vi "Erase color.vi"(8 "error in (no error)":errorcluster, 11 "Control-Client in":refnum<class "Control-Client.lvclass">) -> (0 "error out":errorcluster, 3 "Control-Client out":refnum<class "Control-Client.lvclass">)   [LabVIEW 2015, in "Control-Client.lvclass"]
uses:
  Control-Client.lvclass
  Control-Client.lvclass/Control-Client.ctl
  methods/Read Group #.vi
  Experiments/Experiments_group.lvclass
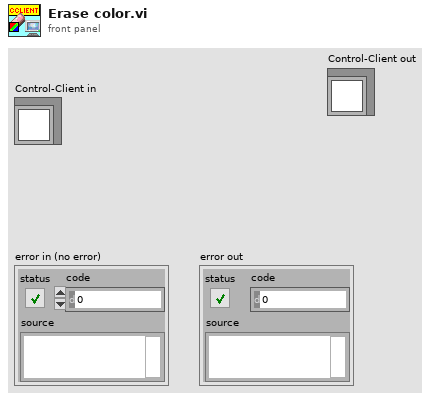
[diagram p1: front panel]
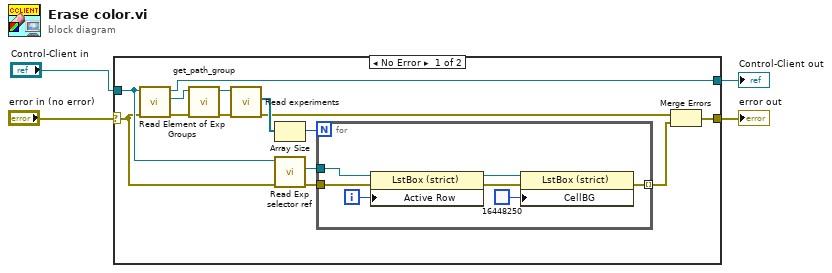
[diagram p0: block diagram]
diagram:
  n1 = case shown="No Error" "error in (no error)" {
    selector: "error in (no error)" -> [w6 w27]
    tunnel: "Control-Client in" -> [w9 w26]
    tunnel: [w7 w26] -> w3
    tunnel: [w5 w27] -> w1
    frame No Error {
      n2 = call "Read Element of Exp Groups.vi"("error in (no error)"=w6, "Control-Client in"=w9) -> ("error out"=w10:errorcluster, "Experiments_group.lvclass"=w11:refnum<class "Experiments_group.lvclass">, "Control-Client out"=w7:refnum<class "Control-Client.lvclass">)  [unwired: 7 in]
      n3 = call "get_path_group.vi"("error in (no error)"=w10, "Experiments_group.lvclass in"=w11) -> ("error out"=w15:errorcluster, "Experiments_group.lvclass out"=w14:refnum<class "Experiments_group.lvclass">)  [unwired: 7 in, 1 out]
      n4 = call "Read experiments.vi"("error in (no error)"=w15, "Experiments_group.lvclass in"=w14) -> ("error out"=w8:errorcluster, "Experiments"=w13:refnum<class "Experiment.lvclass">[])  [unwired: 6 in, 1 out]
      n5 = Array Size(array=w13) -> (size(s)=w12:i32)
      n6 = call "Read Exp selector ref.vi"("error in (no error)"=w6, "Control-Client in"=w9) -> ("error out"=w17:errorcluster, "Exp selector ref"=w16:refnum<vi>)  [unwired: 7 in, 1 out]
      n7 = for {
        N: w12 -> [_]
        tunnel: w16 -> [w24]
        tunnel: w17 -> [w20]
        tunnel: [w19] -> w18 mode=indexing
        i -> [w25]
        n8 = property class="LstBox (strict)"(reference=w24, error in=w20, "Active Row"=w25) -> (reference out=w23:refnum<vi>, error out=w22:errorcluster)
        n9 = property class="LstBox (strict)"(reference=w23, error in=w22, "CellBG"=u32 16448250) -> (error out=w19:errorcluster)  [unwired: 1 out]
      }
      n10 = Merge Errors(w8, w18) -> (w5:errorcluster)
    }
    frame Error {
    }
  }
  "Control-Client out" <- w3
  "error out" <- w1
